vi "OutputData.vi"(8 "error in (no error)":errorcluster, 10 "AppOutputData":variant, 11 "ModuleID":i32) -> (0 "error out":errorcluster)   [LabVIEW 2014, in "AppModule.lvlib"]
uses:
  AppModule.lvlib
  clEventType.ctl
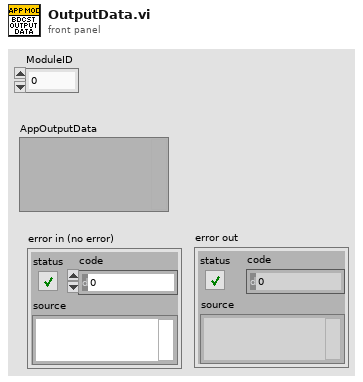
[diagram p1: front panel]
types:
  T1 = typedef "AppModule.lvlib/clEventType.ctl" = cluster{"ModuleID":i32, "Data":variant}
  T2 = typedef "AppModule.lvlib/clBroadcastEvents.ctl" = cluster{"DidInit":refnum<user-event>, "StatusUpdate":refnum<user-event>, "ErrorReport":refnum<user-event>, "DidStop":refnum<user-event>, "PathToINI":refnum<user-event>, "InputData":refnum<user-event>, "OutputData":refnum<user-event>, "BcAppInfo":refnum<user-event>, "ConfigData":refnum<user-event>}
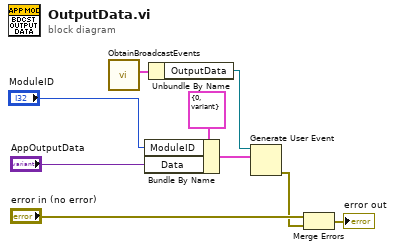
[diagram p0: block diagram]
diagram:
  n1 = call "ObtainBroadcastEvents.vi"() -> ("AppModuleBroadcast"=w7:T2)  [unwired: 10 in, 1 out]
  n2 = Bundle By Name(cluster=T1 {"ModuleID"=0, "Data"=variant} ("clEventType"), "ModuleID"="ModuleID", "Data"="AppOutputData") -> (w6:T1)
  n3 = Unbundle By Name(w7) -> ("OutputData"=w5:refnum<user-event>)
  n4 = Generate User Event(user event=w5, event data cluster=w6) -> (error out=w2:errorcluster)  [unwired: 2 in, 1 out]
  n5 = Merge Errors("error in (no error)", w2) -> (→"error out":errorcluster)
